vi "Vision Follow.vi"(10 "t":T1) -> ()   [LabVIEW 2018]
uses:
  Vision Mode.ctl
  Robot Global Data.vi
  <vilib>/Rock Robotics/Network Tables/NT Read Number.vi
  <vilib>/addons/control/pid/pid.llb/PID (DBL).vi
  <vilib>/addons/control/pid/NI_PID_pid.lvlib
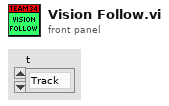
[diagram p1: front panel]
types:
  T1 = typedef "Vision Mode.ctl" = enum16{"Track", "Keep Range", "Follow", "Stop"}
  T2 = typedef "Vision Data.ctl" = cluster{"xOffset":dbl, "yOffset":dbl, "area":dbl, "skewOffset":dbl, "hasTarget":dbl}
  T3 = cluster{"Numeric":dbl, "Numeric":dbl, "Numeric":dbl}
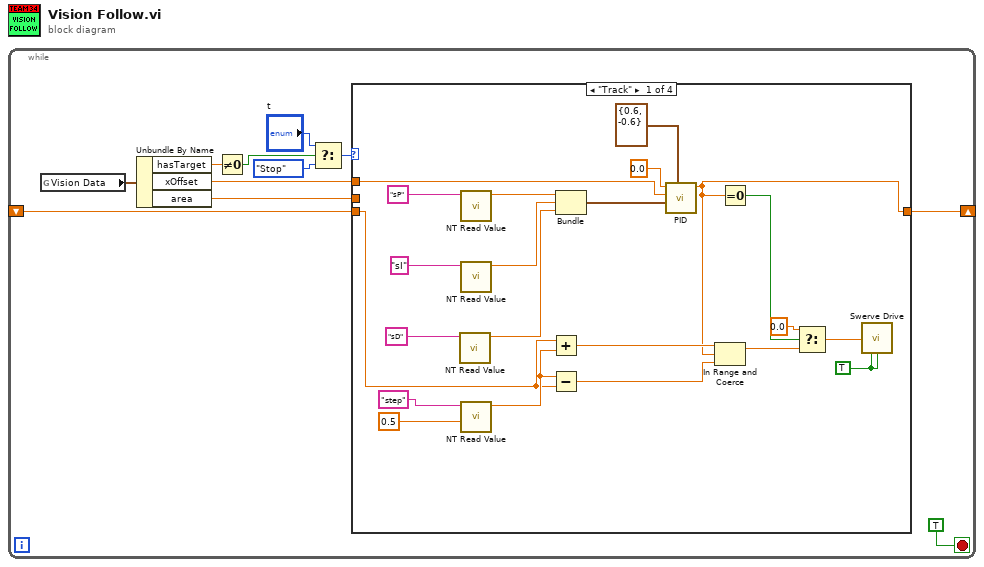
[diagram p0: block diagram]
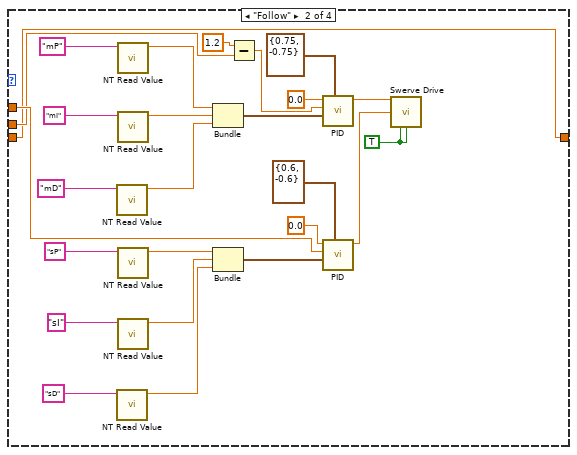
[diagram p2: hidden frame]
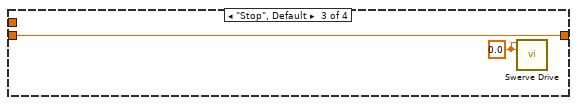
[diagram p3: hidden frame]
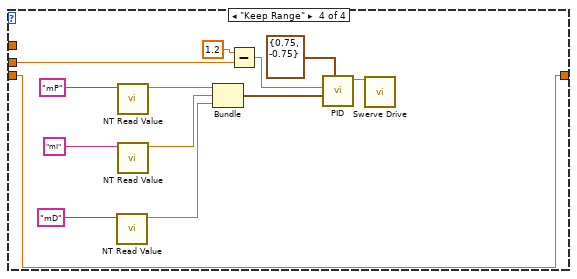
[diagram p4: hidden frame]
diagram:
  n1 = while {
    shift-right: [w2] -> _
    shift-left: _ -> [w1]
    stop <- TRUE stop-if-true
    n2 = global read "Robot Global Data.vi" "Vision Data"() -> (w9:T2)
    n3 = Unbundle By Name(w9) -> ("hasTarget"=w7:dbl, "xOffset"=w8:dbl, "area"=w5:dbl)
    n4 = Not Equal To 0?(x=w7) -> (x != 0?=w6:bool)
    n5 = Select(t="t", s=w6, f=Vision_Mode."Stop" ("Vision Mode")) -> (s? t:f=w10:T1)
    n6 = case shown="\"Track\"" w10 {
      tunnel: w8 -> [w30 w45 _ _]
      tunnel: w5 -> [_ w36 _ w65]
      tunnel: [w13 w34 w60 w62] -> w2
      tunnel: w1 -> [w18 w34 w60 w62]
      frame "Track" {
        w31 = TRUE ("Robot Centric?")
        n7 = call-poly <vilib>:"NT Read Value.vi"("Name"="sD") -> ("Numeric"=w26:dbl)  [unwired: 9 in, 1 out]
        n8 = call-poly <vilib>:"NT Read Value.vi"("Name"="sP") -> ("Numeric"=w24:dbl)  [unwired: 9 in, 1 out]
        n9 = call-poly <vilib>:"NT Read Value.vi"("Name"="sI") -> ("Numeric"=w25:dbl)  [unwired: 9 in, 1 out]
        n10 = call-poly <vilib>:"NT Read Value.vi"("Default Value"=0.5, "Name"="step") -> ("Numeric"=w19:dbl)  [unwired: 8 in, 1 out]
        n11 = Add(x=w18, y=w19) -> (x+y=w20:dbl)
        n12 = Subtract(x=w19, y=w18) -> (x-y=w17:dbl)
        n13 = Bundle("Numeric"=w24, "Numeric"=w25, "Numeric"=w26) -> (w29:T3)  [unwired: 1 in]
        n14 = call-poly <vilib>:"PID.vi"("output range"=cluster{"output high":dbl, "output low":dbl} {"output high"=0.6, "output low"=-0.6}, "PID gains"=w29, "process variable"=w30, "setpoint"=0.0) -> ("output"=w13:dbl)  [unwired: 6 in, 1 out]
        n15 = In Range and Coerce(upper limit=w20, x=w13, lower limit=w17) -> (coerced(x)=w15:dbl)  [unwired: 1 out]
        n16 = Equal To 0?(x=w13) -> (x = 0?=w14:bool)
        n17 = Select(t=0.0, s=w14, f=w15) -> (s? t:f=w16:dbl)
        n18 = call "Swerve Drive.vi"("Z"=w16, "Robot Centric?"=w31, "Autonomous?"=w31) -> ()  [unwired: 8 in, 5 out]
      }
      frame "Follow" {
        w55 = TRUE ("Robot Centric?")
        n19 = call-poly <vilib>:"NT Read Value.vi"("Name"="mD") -> ("Numeric"=w40:dbl)  [unwired: 9 in, 1 out]
        n20 = call-poly <vilib>:"NT Read Value.vi"("Name"="sD") -> ("Numeric"=w50:dbl)  [unwired: 9 in, 1 out]
        n21 = call-poly <vilib>:"NT Read Value.vi"("Name"="mP") -> ("Numeric"=w42:dbl)  [unwired: 9 in, 1 out]
        n22 = call-poly <vilib>:"NT Read Value.vi"("Name"="mI") -> ("Numeric"=w41:dbl)  [unwired: 9 in, 1 out]
        n23 = call-poly <vilib>:"NT Read Value.vi"("Name"="sP") -> ("Numeric"=w48:dbl)  [unwired: 9 in, 1 out]
        n24 = call-poly <vilib>:"NT Read Value.vi"("Name"="sI") -> ("Numeric"=w49:dbl)  [unwired: 9 in, 1 out]
        n25 = Bundle("Numeric"=w42, "Numeric"=w41, "Numeric"=w40) -> (w43:T3)  [unwired: 1 in]
        n26 = Bundle("Numeric"=w48, "Numeric"=w49, "Numeric"=w50) -> (w54:T3)  [unwired: 1 in]
        n27 = Subtract(x=1.2, y=w36) -> (x-y=w37:dbl)
        n28 = call-poly <vilib>:"PID.vi"("output range"=cluster{"output high":dbl, "output low":dbl} {"output high"=0.75, "output low"=-0.75}, "PID gains"=w43, "process variable"=w37, "setpoint"=0.0) -> ("output"=w39:dbl)  [unwired: 6 in, 1 out]
        n29 = call-poly <vilib>:"PID.vi"("output range"=cluster{"output high":dbl, "output low":dbl} {"output high"=0.6, "output low"=-0.6}, "PID gains"=w54, "process variable"=w45, "setpoint"=0.0) -> ("output"=w53:dbl)  [unwired: 6 in, 1 out]
        n30 = call "Swerve Drive.vi"("X"=w39, "Z"=w53, "Robot Centric?"=w55, "Autonomous?"=w55) -> ()  [unwired: 7 in, 5 out]
      }
      frame "Stop", Default {
        w61 = 0.0 ("X")
        n31 = call "Swerve Drive.vi"("X"=w61, "Y"=w61) -> ()  [unwired: 9 in, 5 out]
      }
      frame "Keep Range" {
        n32 = call-poly <vilib>:"NT Read Value.vi"("Name"="mD") -> ("Numeric"=w68:dbl)  [unwired: 9 in, 1 out]
        n33 = call-poly <vilib>:"NT Read Value.vi"("Name"="mP") -> ("Numeric"=w70:dbl)  [unwired: 9 in, 1 out]
        n34 = call-poly <vilib>:"NT Read Value.vi"("Name"="mI") -> ("Numeric"=w69:dbl)  [unwired: 9 in, 1 out]
        n35 = Bundle("Numeric"=w70, "Numeric"=w69, "Numeric"=w68) -> (w71:T3)  [unwired: 1 in]
        n36 = Subtract(x=1.2, y=w65) -> (x-y=w63:dbl)
        n37 = call-poly <vilib>:"PID.vi"("output range"=cluster{"output high":dbl, "output low":dbl} {"output high"=0.75, "output low"=-0.75}, "PID gains"=w71, "process variable"=w63) -> ("output"=w66:dbl)  [unwired: 7 in, 1 out]
        n38 = call "Swerve Drive.vi"("X"=w66) -> ()  [unwired: 10 in, 5 out]
      }
    }
  }
